vi "DecodeSensorBytes.vi"(8 "error in":errorcluster, 11 "VISA resource name":refnum<visa-resource-name>) -> (0 "error out":errorcluster, 3 "VISA resource name out":refnum<visa-resource-name>, 5 "Array":i16[][](array[numeric]), 7 "Bytes":u32)   [LabVIEW 2010]
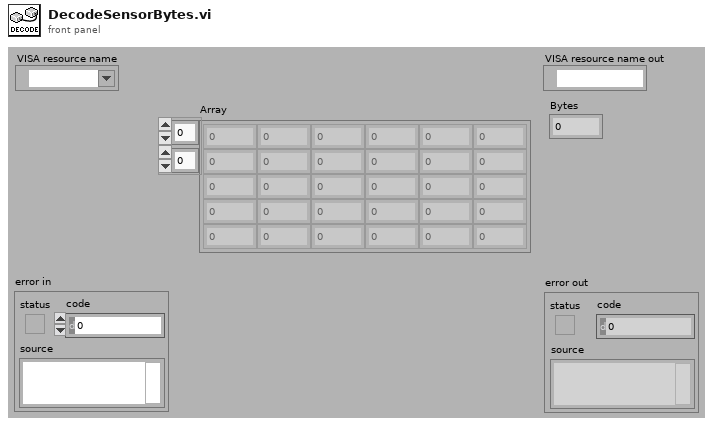
[diagram p1: front panel]
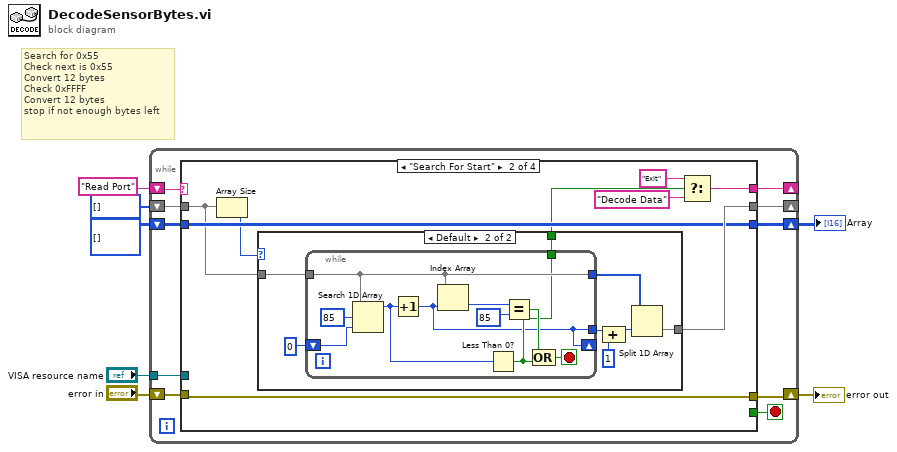
[diagram p0: block diagram]
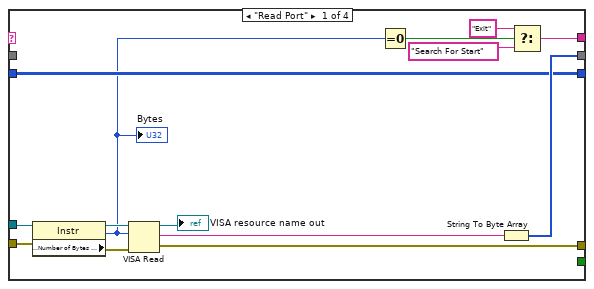
[diagram p2: hidden frame]
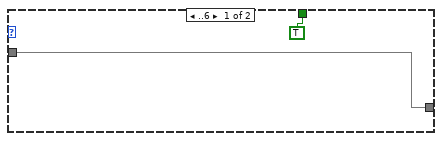
[diagram p3: hidden frame]
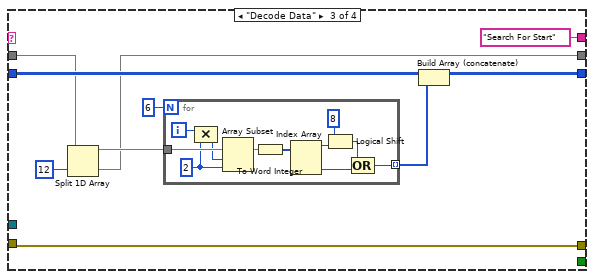
[diagram p4: hidden frame]
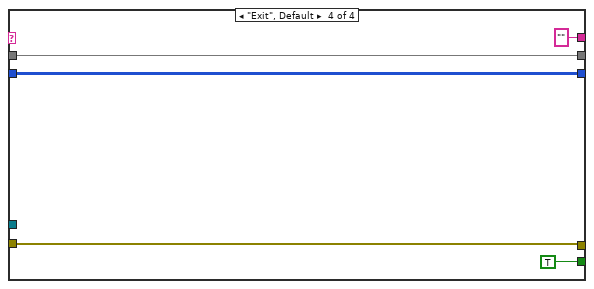
[diagram p5: hidden frame]
diagram:
  # "Search for 0x55\nCheck next is 0x55\nConvert 12 bytes\nCheck 0xFFFF\nConvert 12 bytes\nstop if not enough bytes left"
  n1 = while {
    shift-right: [w12] -> _
    shift-left: "Read Port" -> [w17]
    tunnel: "VISA resource name" -> [w15]
    shift-right: [w13] -> w4
    shift-left: "error in" -> [w14]
    shift-right: [w11] -> _
    shift-left: u8[] [] ("unsigned byte array") -> [w10]
    shift-right: [w8] -> w1
    shift-left: i16[][] [] ("unsigned byte array") -> [w9]
    stop <- w16 stop-if-true
    n2 = case shown="\"Search For Start\"" w17 {
      tunnel: [_ _ _ TRUE] -> w16
      tunnel: w15 -> [w28 _ _ _]
      tunnel: [w25 w40 w63 w85] -> w13
      tunnel: w14 -> [w27 w40 w63 w85]
      tunnel: [w18 w33 "Search For Start" ""] -> w12
      tunnel: [w26 w39 w64 w83] -> w11
      tunnel: w10 -> [_ w37 w65 w83]
      tunnel: w9 -> [w24 w38 w70 w82]
      tunnel: [w24 w38 w68 w82] -> w8
      frame "Read Port" {
        n3 = property class="Instr"(reference=w28, error in=w27) -> (reference out=w30:refnum<visa-resource-name>, error out=w31:errorcluster, "Serial Settings:Number of Bytes at Serial Port"=w19:u32)
        "Bytes" <- w19
        n4 = VISA Read(VISA resource name=w30, byte count=w19, error in (no error)=w31) -> (VISA resource name out=→"VISA resource name out":refnum<visa-resource-name>, read buffer=w29:string, error out=w25:errorcluster)  [unwired: 1 out]
        n5 = Equal To 0?(x=w19) -> (x = 0?=w20:bool)
        n6 = String To Byte Array(string=w29) -> (unsigned byte array=w26:u8[])
        n7 = Select(t="Exit", s=w20, f="Search For Start") -> (s? t:f=w18:string)
      }
      frame "Search For Start" {
        n8 = Array Size(array=w37) -> (size(s)=w36:i32)
        n9 = case shown="Default" w36 {
          tunnel: [w42 w49] -> w39
          tunnel: w37 -> [w42 w48]
          tunnel: [TRUE w44] -> w35
          frame ..6 {
          }
          frame Default {
            n10 = while {
              tunnel: [w51] -> w47
              tunnel: [w58] -> w50
              tunnel: w48 -> [w58]
              tunnel: [w53] -> w44
              shift-right: [w51] -> _
              shift-left: 0 -> [w52]
              stop <- w55 stop-if-true
              n11 = Search 1D Array(1D array=w58, element=u8 85, start index (0)=w52) -> (index of element=w54:i32)
              n12 = Increment(x=w54) -> (x+1=w51:i32)
              n13 = Index Array(array=w58, index=w51) -> (element=w59:u8)
              n14 = Less Than 0?(x=w54) -> (x < 0?=w53:bool)
              n15 = Equal?(x=w59, y=u8 85 ("element")) -> (x = y?=w56:bool)
              n16 = Compound Arithmetic op=OR(w56, w53) -> (w55:bool)
            }
            n17 = Compound Arithmetic op=ADD(w47, 1 ("value")) -> (w46:i32)
            n18 = Split 1D Array(array=w50, index=w46) -> (second subarray=w49:u8[])  [unwired: 1 out]
          }
        }
        n19 = Select(t="Exit", s=w35, f="Decode Data") -> (s? t:f=w33:string)
      }
      frame "Decode Data" {
        n20 = Split 1D Array(array=w65, index=12) -> (first subarray=w66:u8[], second subarray=w64:u8[])
        n21 = for {
          N: 6 -> [_]
          tunnel: [w71] -> w69 mode=indexing
          tunnel: w66 -> [w80]
          i -> [w79]
          w78 = 2 ("length")
          n22 = Compound Arithmetic op=MULTIPLY(w79, w78) -> (w77:i32)
          n23 = Array Subset(array=w80, index=w77, length=w78) -> (w81:u8[])
          n24 = To Word Integer(number=w81) -> (16bit integer=w74:i16[])
          n25 = Index Array(array=w74) -> (element #1=w76:i16, element #2=w73:i16)  [unwired: 2 in]
          n26 = Logical Shift(y=i8 8, x=w76) -> (x << y=w72:i16)
          n27 = Compound Arithmetic op=OR(w72, w73) -> (w71:i16)
        }
        n28 = Build Array (concatenate)(w70, w69) -> (w68:i16[][])
      }
      frame "Exit", Default {
      }
    }
  }
  "error out" <- w4
  "Array" <- w1
